vi "Error 5008 - Invalid PWM Channel Number.vi"() -> (0 "error out":errorcluster)   [LabVIEW 2021]
doc: "Error 5003 - Analog input channel number is invalid."
uses:
  <vilib>/Utility/error.llb/Error Cluster From Error Code.vi
  <vilib>/ErrorRing/Error Ring.xnode
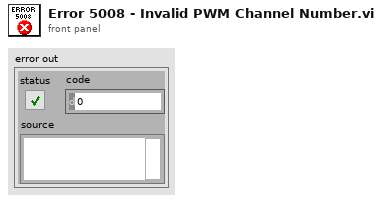
[diagram p1: front panel]
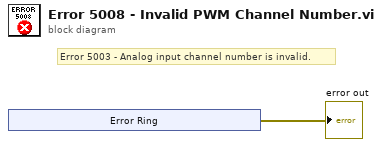
[diagram p0: block diagram]
diagram:
  # "Error 5003 - Analog input channel number is invalid."
  n1 = xnode "Error Ring"() -> ("error out"=→"error out":errorcluster)
